vi "KM_peak -- find -- simple -- V1.vi"(0 "omega in":dbl[](array[numeric]), 1 "z in":cdb[](array[numeric]), 5 "parameters: complex fit":T3={"main VI path"=path "", "scale factor"=3.0, "# of grid points"=200, "parameters: wavepacket"={"R"=0.5, "wave number"=22.0, "delta k"=7.0, "radii vector"=[], "radial section"=[], "wave vector"=22.0, "wavepacket is"=TRUE}, "span"=0.27789, "interference ?"=enum."cp z center", "filter method"=enum."three"} {"span" min=0.0 max=0.5 step=1e-05 scale=0.0001..0.5 scale format="%#_5f"; "parameters: wavepacket"."delta k" format="%#_3f"; "parameters: wavepacket"."wave number" format="%#_3f"; "parameters: wavepacket"."R" format="%#_3f"}, 9 "just guess?":bool, 11 "subtract linear BG":bool) -> (17 "good lorentzian":T1={"Amp (VHz)"=-1.0311345636926572, "f (Hz)"=-1.0311345636926572, "G (Hz)"=-1.0311345636926572, "phi (rad)"=-1.0311345636926572, "Q"=-1.0311345636926572, "Norm  Ampl"=-1.0311345636926572, "bg (V)"=-1.0311345636926572+0.0i, "4corners"={"z (-pi/2)"=-1.0311345636926572+0.5736824521422934i, "z(inf)"=-0.5200164984937075+1.0975277942502903i, "z (pi/2)"=-1.0311345636926572+0.5736824521422934i, "z center"=-0.5136528600391839+0.580046090596817i, "z(0)"=-0.5200164984937075+1.0975277942502903i, "radius"=-1.0311345636926572}} {"bg (V)" format="%#9_9f"; "Q" format="%#9_9f"; "phi (rad)" format="%#9_9f"; "G (Hz)" format="%#9_9f"; "f (Hz)" format="%#9_9f"})   [LabVIEW 2017]
uses:
  peak -- parameters -- complex fit.ctl
  wavepacket.ctl
  filter method control.ctl
  lorentzian.ctl
  circle corners.ctl
  tale of three indices.vi
  Q -- check range -- i -- real.vi
  filter -- window span logic.vi
  linear interp iiii- complex - z-omega - divide.vi
  linear interpolation iiii- complex.vi
  containing bix.vi
  <vilib>/Analysis/baseanly.llb/A x B.vi
  <vilib>/Analysis/baseanly.llb/Complex A x B.vi
  line -- complex.vi
  Q -- check range -- i -- integer.vi
  peak -- guess at omega -- dzdomega V2.vi
  command stack.vi
  tale of three indices -- check state.vi
  Q - not nan -- real.vi
  Q - not nan -- integer.vi
  peak -- z center from mult phase points.vi
  peak -- estimate for lorentzian.vi
  peak -- fake phase around center.vi
  peak -- get weights.vi
  peak -- four corner circle transformation logic.vi
  peak - fit phase around center - V2.vi
  array - generate range.vi
  circle center from three points.vi
  <vilib>/Utility/error.llb/Clear Errors.vi
  <vilib>/gmath/NumericalOptimization/Nonlinear Curve Fit.vi
  <vilib>/gmath/NumericalOptimization/Nonlinear Curve Fit LM.vi
  <vilib>/Analysis/baseanly.llb/Inverse Matrix.vi
  <vilib>/Analysis/baseanly.llb/Real Inverse Matrix.vi
  <vilib>/Analysis/Matrix/Numeric/Conversions/Array To Matrix.vi
  <vilib>/Analysis/Matrix/Numeric/Conversions/Array To Matrix - RA2.vi
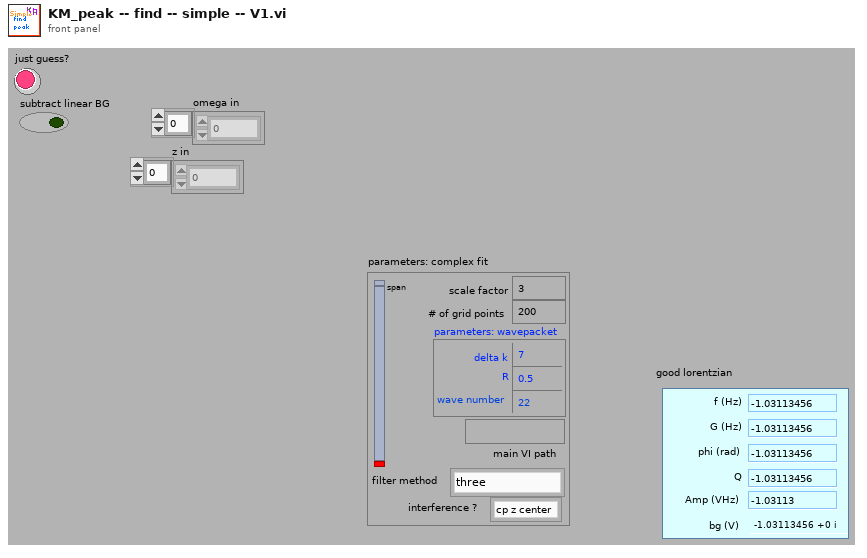
[diagram p1: front panel]
types:
  T1 = typedef "lorentzian.ctl" = cluster{"Amp (VHz)":dbl, "f (Hz)":dbl, "G (Hz)":dbl, "phi (rad)":dbl, "Q":dbl, "Norm  Ampl":dbl, "bg (V)":cdb, "4corners":T2}
  T2 = typedef "circle corners.ctl" = cluster{"z (-pi/2)":cdb, "z(inf)":cdb, "z (pi/2)":cdb, "z center":cdb, "z(0)":cdb, "radius":dbl}
  T3 = typedef "peak -- parameters -- complex fit.ctl" = cluster{"main VI path":path, "scale factor":dbl, "# of grid points":i32, "parameters: wavepacket":T4, "span":dbl, "interference ?":enum16{"cp z center", "pm zcenter", "fancy"}, "filter method":T5}
  T4 = typedef "wavepacket.ctl" = cluster{"R":dbl, "wave number":dbl, "delta k":dbl, "radii vector":dbl[], "radial section":cdb[], "wave vector":dbl, "wavepacket is":bool}
  T5 = typedef "filter method control.ctl" = enum16{"four", "five", "one", "two", "three", "zero", "minus one", "minus two"}
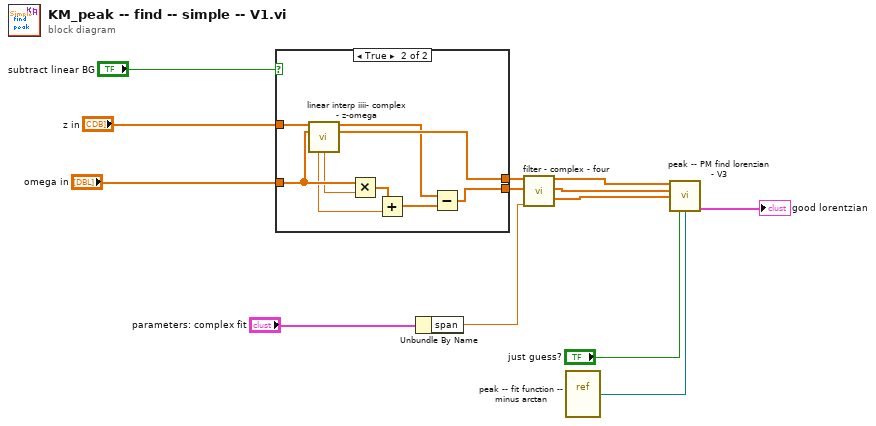
[diagram p0: block diagram]
diagram:
  n1 = case shown="True" "subtract linear BG" {
    tunnel: "omega in" -> [w15 w22]
    tunnel: "z in" -> [w14 w24]
    tunnel: [w14 w16] -> w6
    tunnel: [w15 w23] -> w5
    frame False {
    }
    frame True {
      n2 = call "linear interp iiii- complex - z-omega.vi"("z"=w24, "omega"=w22) -> ("z out"=w18:cdb[], "omega out"=w23:dbl[], "intercept"=w19:cdb, "slope"=w21:cdb)  [unwired: 5 in, 5 out]
      n3 = Multiply(x=w22, y=w21) -> (x*y=w20:cdb[])
      n4 = Add(x=w20, y=w19) -> (x+y=w17:cdb[])
      n5 = Subtract(x=w18, y=w17) -> (x-y=w16:cdb[])
    }
  }
  n6 = Unbundle By Name("parameters: complex fit") -> ("span"=w9:dbl)
  n7 = call "filter - complex - four.vi"("omega  in"=w5, "z in"=w6, "span"=w9) -> ("omega out"=w13:dbl[], "z out"=w11:cdb[], "dz/domega out"=w12:cdb[])  [unwired: 9 in, 5 out]
  n8 = vi-ref "peak -- fit function -- minus arctan.vi"() -> (w1:refnum<vi>)
  n9 = call "peak -- PM find lorenzian - V3.vi"("omega"=w13, "z"=w11, "dz/domega"=w12, "just guess?"="just guess?", "VI Refnum"=w1) -> ("poor man lorentzian"=→"good lorentzian":T1)  [unwired: 7 in, 3 out]
